vi "myRIO v1.0 AI Block Read.vi"(6 "AI FIFO Sample Rate":dbl=1000.0 min=1000.0 max=30000.0, 7 "Scale Constants Array":T1, 8 "error in (no error)":errorcluster, 9 "Number of Samples":u32=1000, 10 "AI (N Samples) Channels List":T3, 11 "myRIO Ref In":T5) -> (0 "error out":errorcluster, 2 "dbl Scaled Value List":dbl[][](array[numeric]), 3 "myRIO Ref Out":T5)   [LabVIEW 2021]
uses:
  <vilib>/myRIO/Common/Instrument Driver Framework/Utilities/typedefs/myRIO v1.0 Reference.ctl
  <vilib>/myRIO/Common/Instrument Driver Framework/Utilities/typedefs/Generic FPGA Reference.ctl
  <vilib>/myRIO/Common/Instrument Driver Framework/myRIO v1.0/AI Block/typedefs/AI Block Channels List.ctl
  <vilib>/myRIO/Common/Instrument Driver Framework/myRIO v1.0/AI Block/typedefs/AI Block Channels Enum.ctl
  <vilib>/myRIO/Common/Instrument Driver Framework/Utilities/typedefs/Analog Scaling Constants List.ctl
  <vilib>/myRIO/Common/Instrument Driver Framework/Utilities/typedefs/Analog Scaling Constants.ctl
  <vilib>/myRIO/Common/Instrument Driver Framework/myRIO v1.0/AI Block/typedefs/AI Block Channels FPGA Reference.ctl
  <vilib>/myRIO/Common/Instrument Driver Framework/myRIO v1.0/Resource Manager/vis/myRIO v1.0 Block Write Configuration.vi
  <vilib>/rvi/errors/niLvFpgaAdjustHostInterfaceError.vi
  <vilib>/rvi/interface/nirviReadWriteControl/nirviReadWriteControl.xnode
  <vilib>/rvi/interface/nirviMethod/nirviMethod.xnode
  <vilib>/rvi/interface/Simulation/niFpgaSimulationCallBeginRW.vi
  <vilib>/rvi/errors/niLvFpgaMergeErrorWithErrorCode.vi
  NiFpgaLv.dll
  <vilib>/FPGAPlugInAG/Dynamic/niLvFpga_StartFifo_Dynamic.vi
  <vilib>/FPGAPlugInAG/Dynamic/niLvFpga_StopFifo_Dynamic.vi
  <vilib>/FPGAPlugInAG/Dynamic/niLvFpga_ReadFifo_Dynamic.vi
panel:
  # "This VI reads a set of analog values from a user specified analog channel on\nthe myRIO v1.0 hardware. The values are read on the FPGA as u16 and \nscaled to dbl based on the specifications of the ADC. Please see Block Diagram for details."
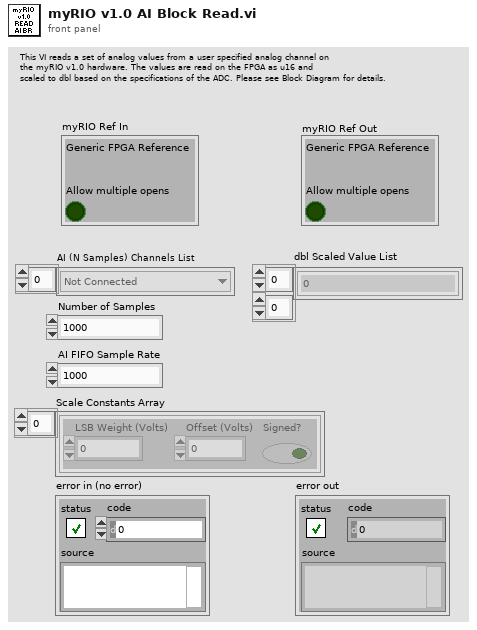
[diagram p1: front panel]
types:
  T1 = typedef "Analog Scaling Constants List.ctl" = T2[]
  T2 = typedef "Analog Scaling Constants.ctl" = cluster{"LSB Weight (Volts)":dbl, "Offset (Volts)":dbl, "Signed?":bool}
  T3 = typedef "AI Block Channels List.ctl" = T4[]
  T4 = typedef "AI Block Channels Enum.ctl" = enum16{"Not Connected", "A/AI0 (N Samples)", "A/AI1 (N Samples)", "A/AI2 (N Samples)", "A/AI3 (N Samples)", "A/AI4 (N Samples)", "A/AI5 (N Samples)", "A/AI6 (N Samples)", "A/AI7 (N Samples)", "A/AI0 (DIFF N Samples)", "A/AI1 (DIFF N Samples)", "A/AI2 (DIFF N Samples)", "A/AI3 (DIFF N Samples)", "B/AI0 (N Samples)", "B/AI1 (N Samples)", "B/AI2 (N Samples)", "B/AI3 (N Samples)", "B/AI4 (N Samples)", "B/AI5 (N Samples)", "B/AI6 (N Samples)", "B/AI7 (N Samples)", "B/AI0 (DIFF N Samples)", "B/AI1 (DIFF N Samples)", "B/AI2 (DIFF N Samples)", "B/AI3 (DIFF N Samples)"}
  T5 = typedef "myRIO v1.0 Reference.ctl" = cluster{"Generic FPGA Reference":T6, "Allow multiple opens":bool}
  T6 = typedef "Generic FPGA Reference.ctl" = refnum<k20>
  T7 = typedef "AI Block Channels FPGA Reference.ctl" = refnum<k20>
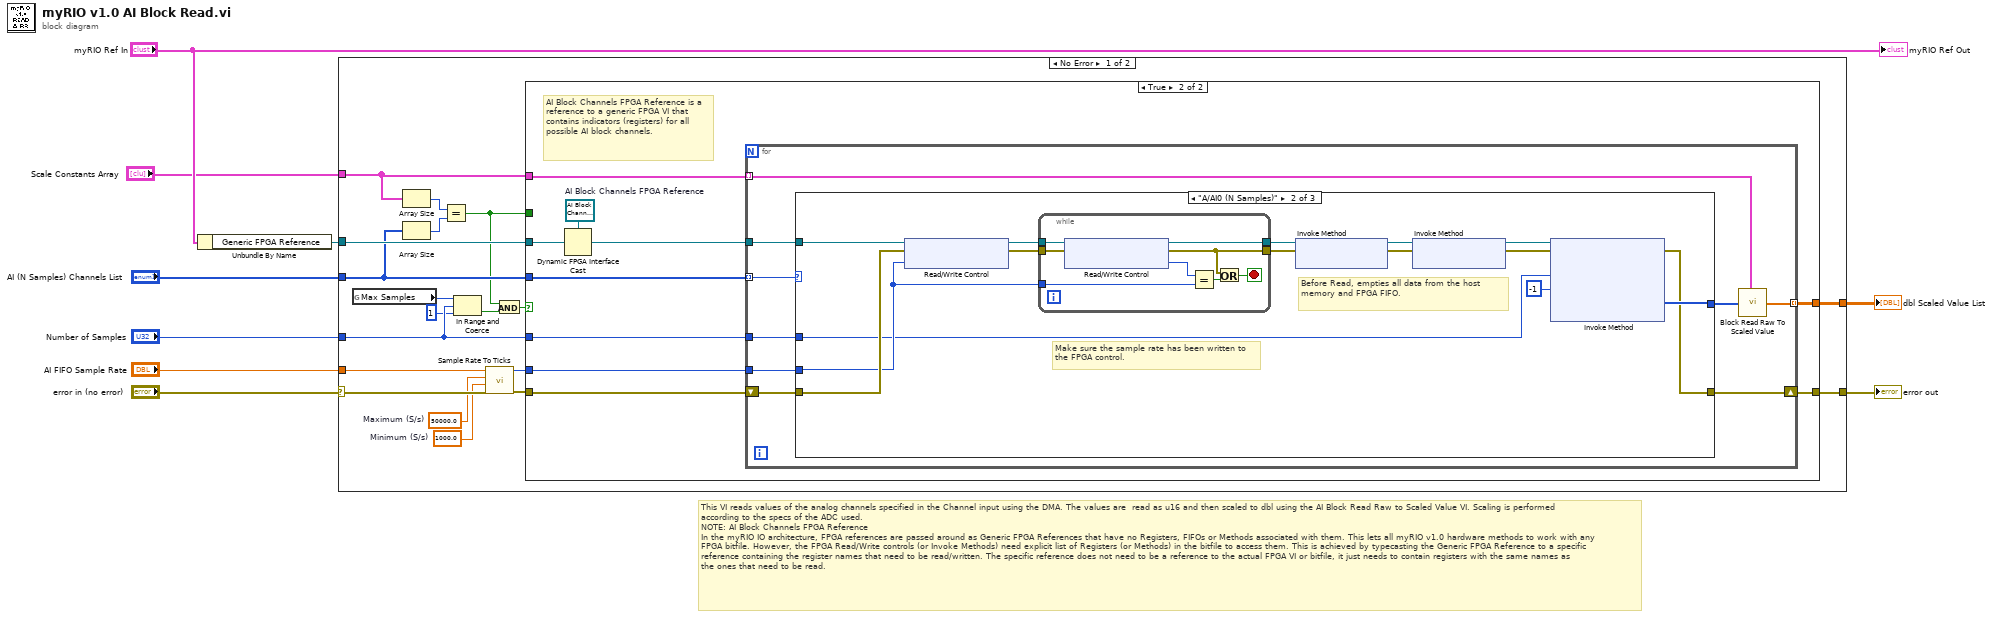
[diagram p0: block diagram]
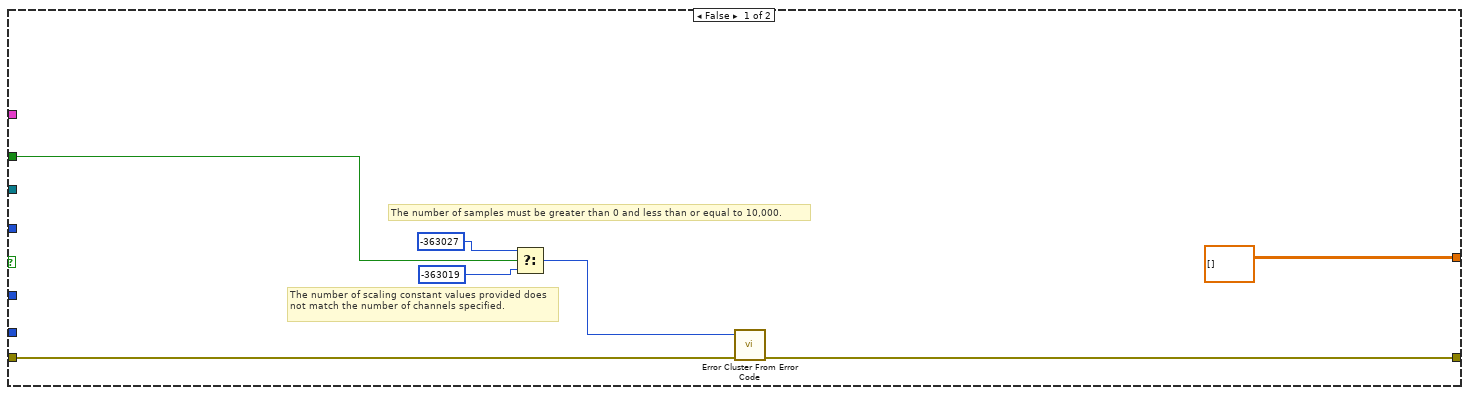
[diagram p2: hidden frame]
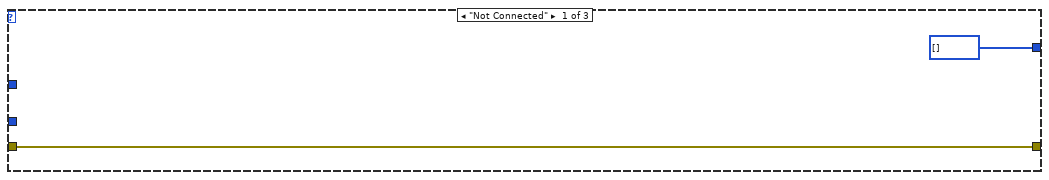
[diagram p3: hidden frame]
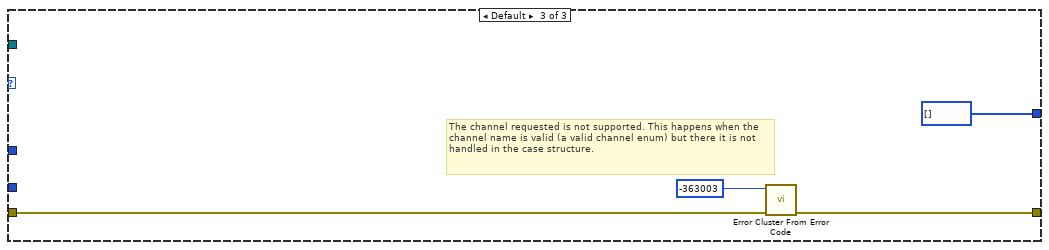
[diagram p4: hidden frame]
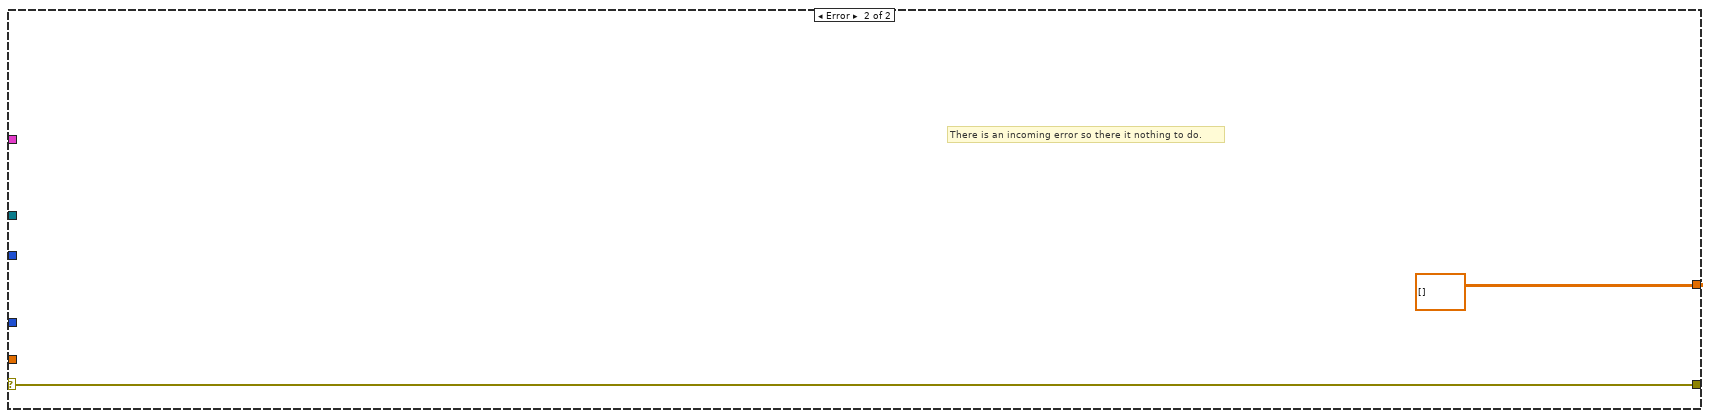
[diagram p5: hidden frame]
diagram:
  # "This VI reads values of the analog channels specified in the Channel input using the DMA. The values are  read as u16 and then scaled to dbl using the AI Block Read Raw to Scaled Value VI. Scaling is performed according to the specs of the ADC used.\nNOTE: AI Block Channels FPGA Reference\nIn the myRIO IO architecture, FPGA references are passed around as Generic FPGA References that have no Registers, FIFOs or Methods associated with them. This lets all myRIO v1.0 hardware methods to work with any FPGA bitfile. However, the FPGA Read/Write controls (or Invoke Methods) need explicit list of Registers (or Methods) in the bitfile to access them. This is achieved by typecasting the Generic FPGA Reference to a specific reference containing the register names that need to be read/written. The specific reference does not need to be a reference to the actual FPGA VI or bitfile, it just needs to contain registers with the same names as the ones that need to be read."
  n1 = Unbundle By Name("myRIO Ref In") -> ("Generic FPGA Reference"=w6:T6)
  n2 = case shown="No Error" "error in (no error)" {
    selector: "error in (no error)" -> [w18 w85]
    tunnel: w6 -> [w28 _]
    tunnel: [w27 w85] -> w9
    tunnel: [w26 dbl[][] [] ("dbl Scaled Value")] -> w8
    tunnel: "AI (N Samples) Channels List" -> [w23 _]
    tunnel: "AI FIFO Sample Rate" -> [w19 _]
    tunnel: "Number of Samples" -> [w12 _]
    tunnel: "Scale Constants Array" -> [w22 _]
    frame No Error {
      w14 = 1000.0  # Minimum (S/s)
      w15 = 50000.0  # Maximum (S/s)
      n3 = global read "myRIO v1.0 Block Write Configuration.vi" "Max Samples"() -> (w13:u32)
      n4 = Array Size(array=w22) -> (size(s)=w24:i32)
      n5 = Array Size(array=w23) -> (size(s)=w25:i32)
      n6 = Equal?(x=w24, y=w25) -> (x = y?=w20:bool)
      n7 = In Range and Coerce(upper limit=w13, x=w12, lower limit=u32 1) -> (In Range?=w10:bool)  [unwired: 1 out]
      n8 = call <vilib>:"Sample Rate To Ticks.vi"("error in (no error)"=w18, "Minimum (S/s)"=w14, "Maximum (S/s)"=w15, "Sample Rate (S/s)"=w19) -> ("error out"=w16:errorcluster, "Count (tick/s)"=w17:u32)  [unwired: 5 in, 1 out]
      n9 = And(x=w20, y=w10) -> (x .and. y?=w21:bool)
      n10 = case shown="True" w21 {
        tunnel: w28 -> [_ w45]
        tunnel: [w34 w44] -> w27
        tunnel: w16 -> [w35 w43]
        tunnel: [dbl[][] [] ("dbl Scaled Value") w42] -> w26
        tunnel: w17 -> [_ w41]
        tunnel: w12 -> [_ w40]
        tunnel: w23 -> [_ w37]
        tunnel: w22 -> [_ w36]
        tunnel: w20 -> [w32 _]
        frame False {
          # "The number of samples must be greater than 0 and less than or equal to 10,000."
          # "The number of scaling constant values provided does not match the number of channels specified."
          n11 = Select(t=-363027 ("error code (0)"), s=w32, f=-363019 ("error code (0)")) -> (s? t:f=w31:i32)
          n12 = call <vilib>:"Error Cluster From Error Code.vi"("error in (no error)"=w35, "error code (0)"=w31) -> ("error out"=w34:errorcluster)  [unwired: 7 in]
        }
        frame True {
          w39 = T7 refnum  # AI Block Channels FPGA Reference
          # "AI Block Channels FPGA Reference is a reference to a generic FPGA VI that contains indicators (registers) for all possible AI block channels."
          n13 = Dynamic FPGA Interface Cast(Session In=w39, Type=w45) -> (Session Out=w38:T7)
          n14 = for {
            tunnel: w38 -> [w54]
            shift-right: [w52] -> w44
            shift-left: w43 -> [w53]
            tunnel: w37 -> [w51] mode=indexing
            tunnel: [w49] -> w42 mode=indexing
            tunnel: w40 -> [w48]
            tunnel: w41 -> [w47]
            tunnel: w36 -> [w46] mode=indexing
            n15 = case shown="\"A/AI0 (N Samples)\"" w51 {
              tunnel: w53 -> [w56 w67 w81]
              tunnel: [w56 w57 w82] -> w52
              tunnel: [u16[] [] ("Data") w58 u16[] [] ("Data")] -> w50
              tunnel: w54 -> [_ w71 _]
              tunnel: w48 -> [_ w60 _]
              tunnel: w47 -> [_ w66 _]
              frame "Not Connected" {
              }
              frame "A/AI0 (N Samples)" {
                # "Make sure the sample rate has been written to the FPGA control."
                # "Before Read, empties all data from the host memory and FPGA FIFO."
                n16 = xnode "Read/Write Control"("FPGA VI Reference In"=w71, "error in"=w67, "AI.A_0.SampleRate"=w66) -> ("FPGA VI Reference Out"=w69:T7, "error out"=w68:errorcluster)
                n17 = while {
                  tunnel: w69 -> [w76]
                  tunnel: w68 -> [w75]
                  tunnel: [w74] -> w70
                  tunnel: [w73] -> w61
                  tunnel: w66 -> [w79]
                  stop <- w77 stop-if-true
                  n18 = xnode "Read/Write Control"("FPGA VI Reference In"=w76, "error in"=w75) -> ("FPGA VI Reference Out"=w74:T7, "error out"=w73:errorcluster, "AI.A_0.SampleRate"=w72:u32)
                  n19 = Equal?(x=w72, y=w79) -> (x = y?=w78:bool)
                  n20 = Or(x=w73, y=w78) -> (x .or. y?=w77:bool)
                }
                n21 = xnode "Invoke Method"("FPGA VI Reference In"=w70, "error in"=w61) -> ("FPGA VI Reference Out"=w65:T7, "error out"=w62:errorcluster)
                n22 = xnode "Invoke Method"("FPGA VI Reference In"=w65, "error in"=w62) -> ("FPGA VI Reference Out"=w64:T7, "error out"=w63:errorcluster)
                n23 = xnode "Invoke Method"("FPGA VI Reference In"=w64, "error in"=w63, "Number of Elements"=w60, "Timeout (ms)"=-1) -> ("error out"=w57:errorcluster, "Data"=w58:u16[])  [unwired: 2 out]
              }
              frame Default {
                # "The channel requested is not supported. This happens when the channel name is valid (a valid channel enum) but there it is not handled in the case structure."
                n24 = call <vilib>:"Error Cluster From Error Code.vi"("error in (no error)"=w81, "error code (0)"=-363003) -> ("error out"=w82:errorcluster)  [unwired: 7 in]
              }
            }
            n25 = call <vilib>:"Block Read Raw To Scaled Value.vi"("Scaling Constants"=w46, "u16 Raw Value"=w50) -> ("dbl Scaled Value"=w49:dbl[])  [unwired: 7 in]
          }
        }
      }
    }
    frame Error {
      # "There is an incoming error so there it nothing to do."
    }
  }
  "error out" <- w9
  "dbl Scaled Value List" <- w8
  "myRIO Ref Out" <- "myRIO Ref In"
